vi "总氮启动流程.vi"() -> ()   [LabVIEW 2016]
uses:
  <vilib>/Utility/miscctls.llb/LVPointTypeDef.ctl
panel:
  out "加标回收实测值":sgl
  out "加标回收数据时间":timestamp
  out "跨度核查实测值":sgl
  out "跨度核查数据时间":timestamp
  out "空白实测值":sgl
  out "空白数据时间":timestamp
  out "水样实测值":sgl
  out "水样数据时间":timestamp
  out "启动记录":string
  out "流程运行中":bool
  out "启动次数":i32
  out "日期/时间":string
  out "运行状态":string
  out "步骤运行时间/秒":i32
  out "流程结束":bool
  out "当前步骤":T1(ring)
  in  "步骤时间/秒":T2={"步骤1时间"=2, "步骤2时间"=4, "步骤3时间"=2, "步骤4时间"=5, "步骤5时间"=6, "步骤6时间"=3, "步骤7时间"=4, "步骤8时间"=7, "步骤9时间"=8, "步骤10时间"=6}
  # "总氮模块"
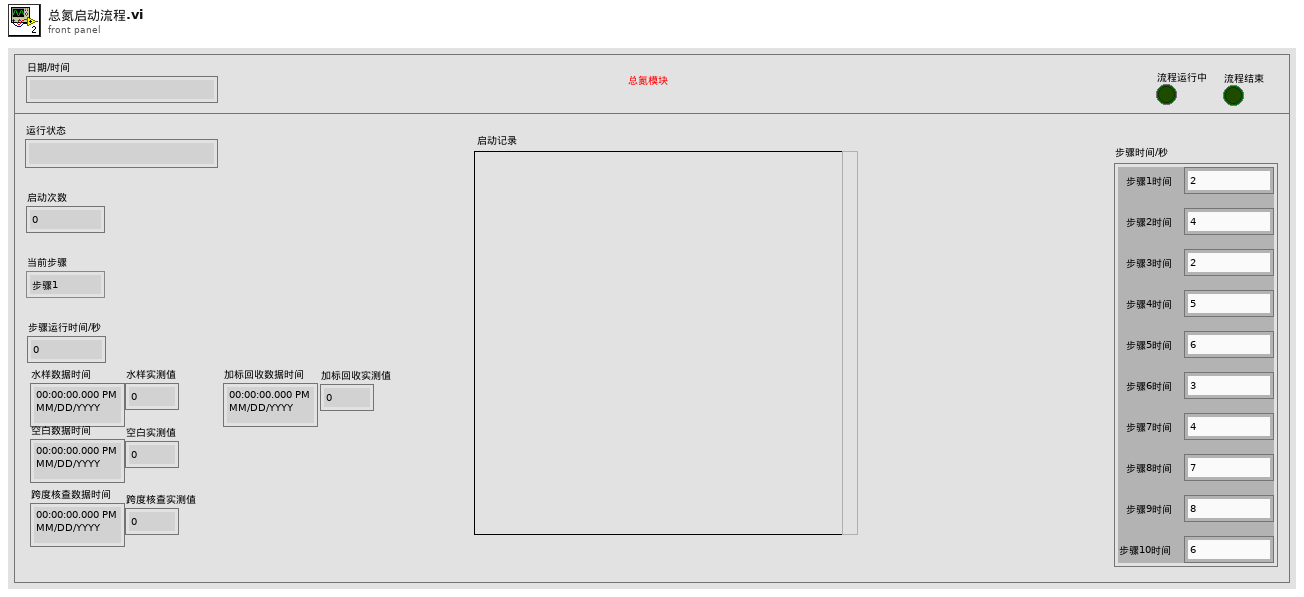
[diagram p1: front panel]
types:
  T1 = enum16{"步骤1", "步骤2", "步骤3", "步骤4", "步骤5", "步骤6", "步骤7", "步骤8", "步骤9", "步骤10"}
  T2 = cluster{"步骤1时间":i32, "步骤2时间":i32, "步骤3时间":i32, "步骤4时间":i32, "步骤5时间":i32, "步骤6时间":i32, "步骤7时间":i32, "步骤8时间":i32, "步骤9时间":i32, "步骤10时间":i32}
  T3 = enum16{"write register", "read register", "write and read register", "write coil", "read coil"}
  T4 = typedef "LVPointTypeDef.ctl" = cluster{"Horizontal":i16, "Vertical":i16}
  T5 = enum32{"Bad", "Idle", "Run top level", "Running"}
  T6 = cluster{"系统时间":timestamp, "工作状态":u16, "测量模式":u16, "告警代码":enum16{"无告警", "缺试剂告警", "缺水样告警", "缺蒸馏水告警", "缺标液告警", "仪表漏液告警", "标定异常告警", "超量程告警", "加热异常", "低试剂预警", "超上限告警", "超下限告警", "仪表内部其他异常", "滴定异常告警", "电极异常告警", "量程切换告警", "参数设置告警", "PH电极电位异常", "电导率电极异常", "浊度光度异常", "溶解氧电极异常", "溶解氧光强异常", "温度异常告警", "PH异常告警", "溶解氧异常告警", "电导率异常告警", "浊度异常告警", "叶绿素异常告警", "藻密度异常告警", "蓝绿藻异常告警", "ORP异常告警", "氨氮异常告警", "清洁刷异常告警", "SD卡异常告警", "蓝牙异常告警", "Wifi异常告警", "流程异常告警"}, "故障代码":enum16{"无故障", "电机故障", "温度故障", "通讯故障", "滴定故障"}, "日志代码":u16, "软件版本":u16, "F0":sgl, "F1":sgl, "F2":sgl, "F3":sgl, "T":sgl, "H":sgl, "id":u16, "flowid":u16, "量程":u16}
  T7 = cluster{"因子编码":u32, "单位":u16, "标样参考值":sgl, "水样数据时间":timestamp, "水样实测值":sgl, "水样数据标识":string, "标样数据时间":timestamp, "标样实测值":sgl, "标样数据标识":string, "空白数据时间":timestamp, "空白实测值":sgl, "空白数据标识":string, "零点核查数据时间":timestamp, "零点核查实测值":sgl, "零点核查数据标识":string, "跨度核查数据时间":timestamp, "跨度核查实测值":sgl, "跨度核查数据标识":string, "加标回收数据时间":timestamp, "加标回收实测值":sgl, "加标回收数据标识":string, "平行样数据时间":timestamp, "平行样实测值":sgl, "平行样数据标识":string}
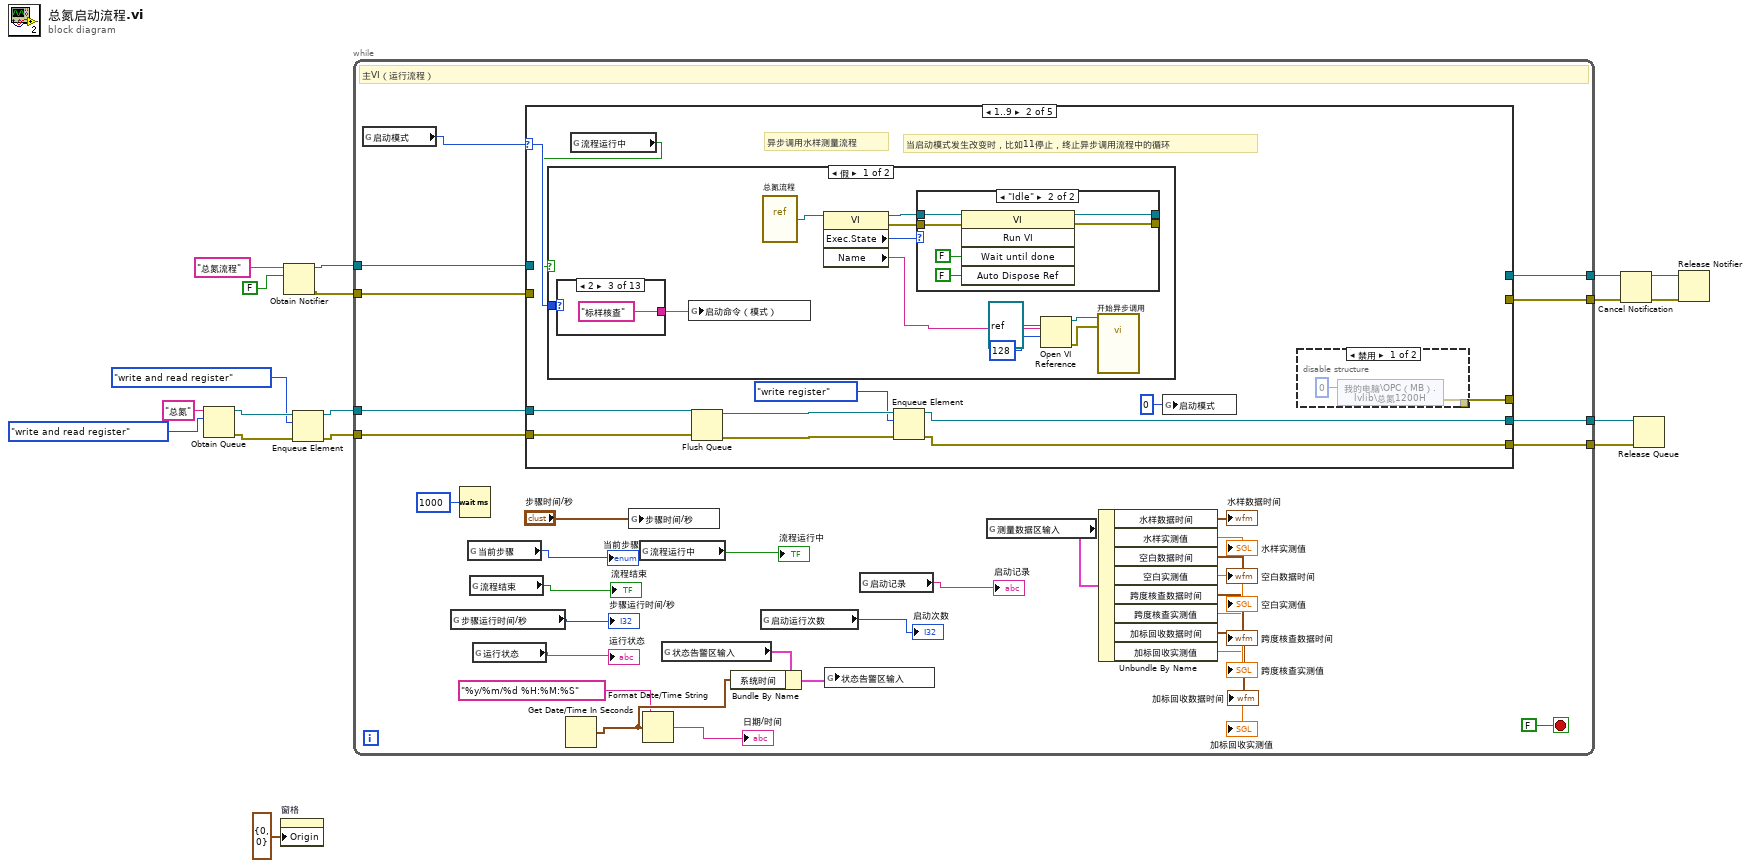
[diagram p0: block diagram]
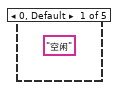
[diagram p2: hidden frame]
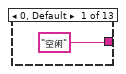
[diagram p4: hidden frame]
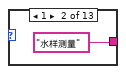
[diagram p5: hidden frame]
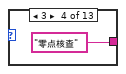
[diagram p6: hidden frame]
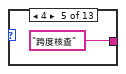
[diagram p7: hidden frame]
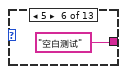
[diagram p8: hidden frame]
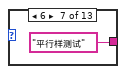
[diagram p9: hidden frame]
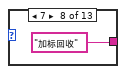
[diagram p10: hidden frame]
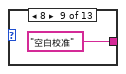
[diagram p11: hidden frame]
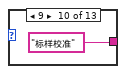
[diagram p12: hidden frame]
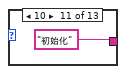
[diagram p13: hidden frame]
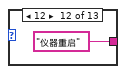
[diagram p14: hidden frame]
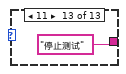
[diagram p15: hidden frame]
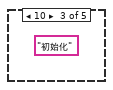
[diagram p18: hidden frame]
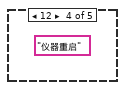
[diagram p19: hidden frame]
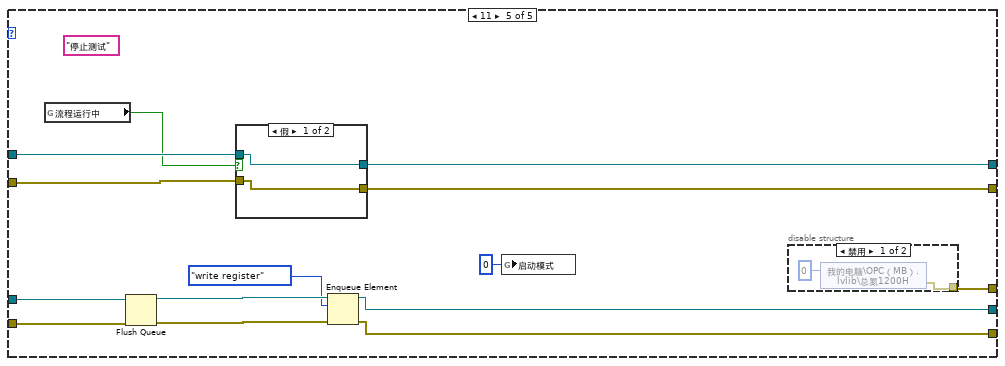
[diagram p20: hidden frame]
diagram:
  n1 = Obtain Queue(name (unnamed)="总氮" ("名称（未命名）"), element data type=T3."write and read register") -> (queue out=w7:refnum<queue>, error out=w6:errorcluster)  [unwired: 3 in, 1 out]
  n2 = property on="窗格" class="Pane"("Origin"=T4 {"Horizontal"=0, "Vertical"=0} ("原点")) -> ()  [unwired: 2 in, 2 out]
  n3 = Obtain Notifier(name (unnamed)="总氮流程" ("名称（未命名）"), notification data type=FALSE) -> (notifier out=w14:refnum<notifier>, error out=w13:errorcluster)  [unwired: 2 in, 1 out]
  n4 = Enqueue Element(queue=w7, element=T3."write and read register", error in (no error)=w6) -> (queue out=w4:refnum<queue>, error out=w3:errorcluster)  [unwired: 1 in, 1 out]
  n5 = while {
    tunnel: w13 -> [w49]
    tunnel: w14 -> [w48]
    tunnel: [w47] -> w17
    tunnel: [w46] -> w18
    tunnel: w4 -> [w32]
    tunnel: w3 -> [w31]
    tunnel: [w30] -> w2
    tunnel: [w29] -> w1
    stop <- FALSE stop-if-true
    # "主VI（运行流程）"
    n6 = global read "总氮全局.vi" "启动模式"() -> (w19:u16)
    n7 = global read "总氮全局.vi" "步骤运行时间/秒"() -> (→"步骤运行时间/秒":i32)
    n8 = Wait (ms)(milliseconds to wait=u32 1000 ("等待时间（毫秒）")) -> ()  [unwired: 1 out]
    n9 = global read "总氮全局.vi" "当前步骤"() -> (→"当前步骤":T1)
    n10 = global read "总氮全局.vi" "流程结束"() -> (→"流程结束":bool)
    n11 = global read "总氮全局.vi" "运行状态"() -> (→"运行状态":string)
    n12 = case shown="1..9" w19 {
      selector: w19 -> [_ w62 _ _ _]
      tunnel: w49 -> [_ _ _ _ w110]
      tunnel: w48 -> [_ _ _ _ w109]
      tunnel: [_ _ _ _ w108] -> w47
      tunnel: [_ _ _ _ w107] -> w46
      tunnel: w32 -> [_ w58 _ _ w103]
      tunnel: w31 -> [_ w57 _ _ w102]
      tunnel: [_ w56 _ _ w101] -> w30
      tunnel: [_ w55 _ _ w100] -> w29
      tunnel: [_ w53 _ _ w98] -> _
      frame 0, Default {
        (unwired) "空闲"
      }
      frame 1..9 {
        # "当启动模式发生改变时，比如11停止，终止异步调用流程中的循环"
        # "异步调用水样测量流程"
        n13 = global read "总氮全局.vi" "流程运行中"() -> (w54:bool)
        n14 = case shown="假" w54 {
          tunnel: w62 -> [w66 _]
          frame False {
            n15 = case shown="2" w66 {
              tunnel: ["空闲" "水样测量" "标样核查" "零点核查" "跨度核查" "空白测试" "平行样测试" "加标回收" "空白校准" "标样校准" "初始化" "仪器重启" "停止测试"] -> w65
              frame 0, Default {
              }
              frame 1 {
              }
              frame 2 {
              }
              frame 3 {
              }
              frame 4 {
              }
              frame 5 {
              }
              frame 6 {
              }
              frame 7 {
              }
              frame 8 {
              }
              frame 9 {
              }
              frame 10 {
              }
              frame 12 {
              }
              frame 11 {
              }
            }
            n16 = global write "总氮全局.vi" "启动命令（模式）"(w65) -> ()
            n17 = vi-ref "总氮流程.vi"() -> (w75:refnum<vi>)
            n18 = property class="VI"(reference=w75) -> (reference out=w74:refnum<vi>, error out=w72:errorcluster, "Exec.State"=w73:T5, "Name"=w67:string)  [unwired: 1 in]
            n19 = case shown="\"Idle\"" w73 {
              tunnel: w74 -> [w90 w96]
              tunnel: [w90 w95] -> _
              tunnel: w72 -> [w89 w92]
              tunnel: [w89 w91] -> _
              frame "Bad", Default {
              }
              frame "Idle" {
                n20 = invoke class="VI" method="Run VI"(reference=w96, error in=w92, "Wait until done"=FALSE ("结束前等待"), "Auto Dispose Ref"=FALSE ("自动销毁引用")) -> (reference out=w95:refnum<vi>, error out=w91:errorcluster)  [unwired: 1 in, 3 out]
              }
            }
            n21 = Open VI Reference(type specifier VI Refnum (for type only)=refnum<vi> refnum ("类型说明符VI引用句柄（仅用于类型）"), vi path=w67, options=128 ("选项")) -> (vi reference=w71:refnum<vi>, error out=w69:errorcluster)  [unwired: 3 in]
            n22 = call-by-ref "开始异步调用"(reference=w71, error in=w69) -> ()  [unwired: 12 in, 2 out]
          }
          frame True {
          }
        }
        n23 = Flush Queue(queue=w58, error in (no error)=w57) -> (queue out=w61:refnum<queue>, error out=w60:errorcluster)  [unwired: 1 out]
        n24 = Enqueue Element(queue=w61, element=T3."write register", error in (no error)=w60) -> (queue out=w56:refnum<queue>, error out=w55:errorcluster)  [unwired: 1 in, 1 out]
        n25 = global write "总氮全局.vi" "启动模式"(u16 0 ("启动模式")) -> ()
        n26 = disable-structure shown="禁用" {
          disable-tunnel: [w63 _] -> w53
          frame Disabled {
            n27 = shared-variable "我的电脑\\OPC（MB）.lvlib\\总氮1200H"(u16 0 ("总氮1200H")) -> (error out=w63:errorcluster)  [unwired: 1 in]
          }
          frame Enabled {
          }
        }
      }
      frame 10 {
        (unwired) "初始化"
      }
      frame 12 {
        (unwired) "仪器重启"
      }
      frame 11 {
        (unwired) "停止测试"
        n28 = global read "总氮全局.vi" "流程运行中"() -> (w99:bool)
        n29 = Flush Queue(queue=w103, error in (no error)=w102) -> (queue out=w106:refnum<queue>, error out=w105:errorcluster)  [unwired: 1 out]
        n30 = case shown="假" w99 {
          tunnel: w110 -> [w113 w118]
          tunnel: w109 -> [w114 w117]
          tunnel: [w114 w116] -> w108
          tunnel: [w113 w115] -> w107
          frame False {
          }
          frame True {
            n31 = Send Notification(notification=TRUE ("通知"), notifier=w117, error in (no error)=w118) -> (notifier out=w116:refnum<notifier>, error out=w115:errorcluster)
          }
        }
        n32 = Enqueue Element(queue=w106, element=T3."write register", error in (no error)=w105) -> (queue out=w101:refnum<queue>, error out=w100:errorcluster)  [unwired: 1 in, 1 out]
        n33 = global write "总氮全局.vi" "启动模式"(u16 0 ("启动模式")) -> ()
        n34 = disable-structure shown="禁用" {
          disable-tunnel: [w111 _] -> w98
          frame Disabled {
            n35 = shared-variable "我的电脑\\OPC（MB）.lvlib\\总氮1200H"(u16 0 ("总氮1200H")) -> (error out=w111:errorcluster)  [unwired: 1 in]
          }
          frame Enabled {
          }
        }
      }
    }
    n36 = Get Date/Time In Seconds() -> (seconds since 1Jan1904=w45:timestamp)
    n37 = global write "总氮全局.vi" "步骤时间/秒"("步骤时间/秒") -> ()
    n38 = global read "总氮全局.vi" "流程运行中"() -> (→"流程运行中":bool)
    n39 = Format Date/Time String(time format string (%c)="%y/%m/%d %H:%M:%S" ("时间格式字符串(%c)"), seconds (now)=w45) -> (date/time string=→"日期/时间":string)  [unwired: 1 in]
    n40 = global read "总氮全局.vi" "状态告警区输入"() -> (w41:T6)
    n41 = Bundle By Name(cluster=w41, "系统时间"=w45) -> (w40:T6)
    n42 = global read "总氮全局.vi" "启动运行次数"() -> (→"启动次数":i32)
    n43 = global write "总氮全局.vi" "状态告警区输入"(w40) -> ()
    n44 = global read "总氮全局.vi" "启动记录"() -> (→"启动记录":string)
    n45 = global read "总氮全局.vi" "测量数据区输入"() -> (w28:T7)
    n46 = Unbundle By Name(w28) -> ("水样数据时间"=→"水样数据时间":timestamp, "水样实测值"=→"水样实测值":sgl, "空白数据时间"=→"空白数据时间":timestamp, "空白实测值"=→"空白实测值":sgl, "跨度核查数据时间"=→"跨度核查数据时间":timestamp, "跨度核查实测值"=→"跨度核查实测值":sgl, "加标回收数据时间"=→"加标回收数据时间":timestamp, "加标回收实测值"=→"加标回收实测值":sgl)
  }
  n47 = Cancel Notification(0:w17, 3:w18) -> (8:w16:refnum<notifier>, 11:w15:errorcluster)  [unwired: 1 out]
  n48 = Release Queue(queue=w2, error in (no error)=w1) -> ()  [unwired: 1 in, 3 out]
  n49 = Release Notifier(notifier=w16, error in (no error)=w15) -> ()  [unwired: 1 in, 3 out]
